vi "GOOP_MyComputer_Item_OnCommand.vi"(10 "Command Tag":string, 11 "Object":u64) -> ()   [LabVIEW 2012]
uses:
  <resource>/Framework/Providers/Open_GDS/SubVIs/GOOP_UMLEditor_CallMainAction.ctl
  <resource>/Framework/Providers/Open_GDS/ClassProviders/Provider_BaseClassInterface/ClassWriter_class/ClassWriter.lvclass
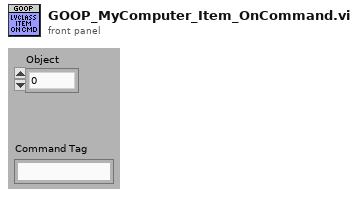
[diagram p1: front panel]
types:
  T1 = typedef "GOOP_UMLEditor_CallMainAction.ctl" = enum16{"OpenUmlEditor", "ReverseEngineering:WholeProject", "ReverseEngineering:OneClass", "ReverseEngineering:OneVI", "ShowInStateDiagram:OneVI", "OpenUMLFile"}
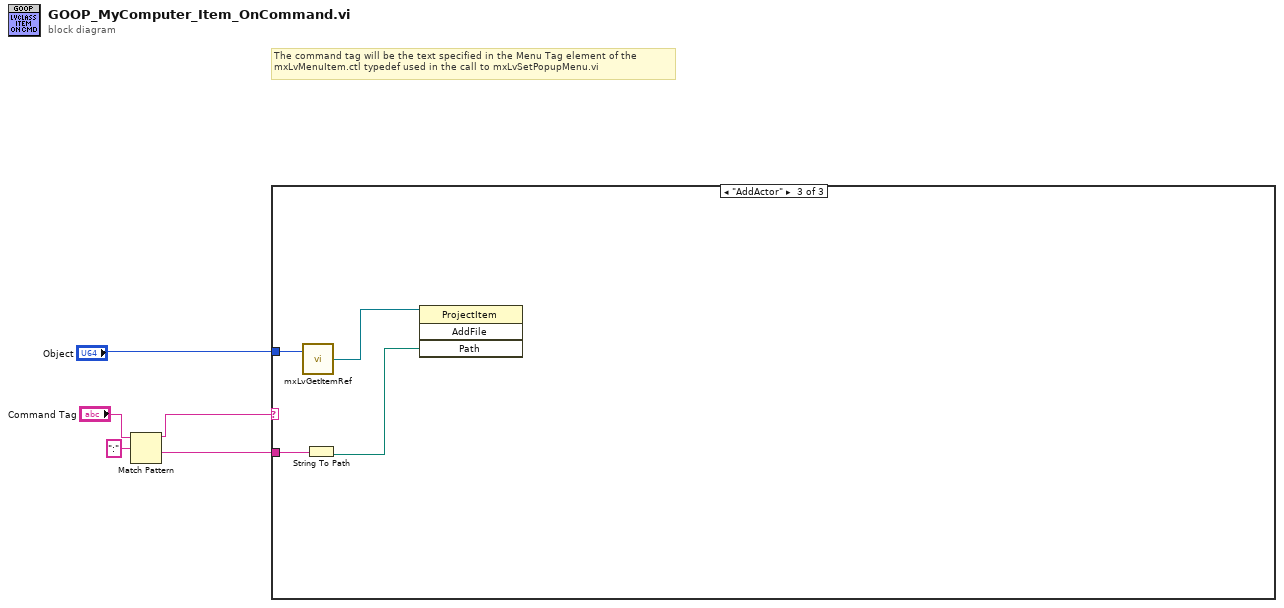
[diagram p0: block diagram]
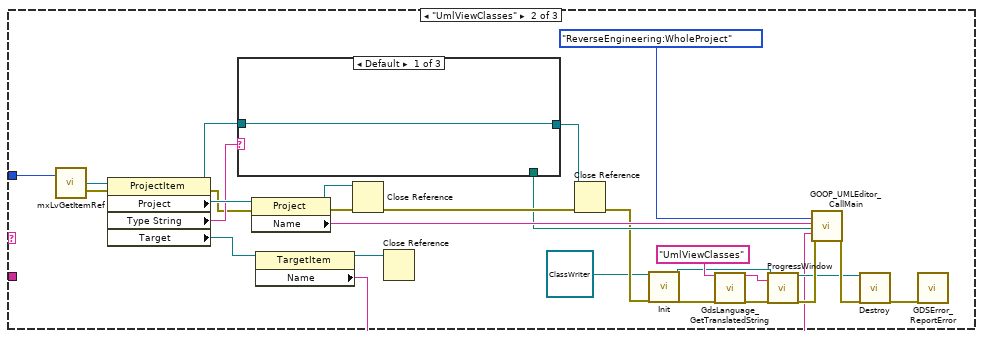
[diagram p3: hidden frame]
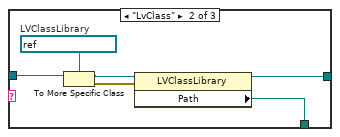
[diagram p4: hidden frame]
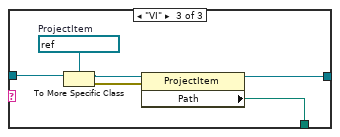
[diagram p5: hidden frame]
diagram:
  # "The command tag will be the text specified in the Menu Tag element of the \nmxLvMenuItem.ctl typedef used in the call to mxLvSetPopupMenu.vi"
  n1 = Match Pattern(string="Command Tag", regular expression=":") -> (before substring=w2:string, after substring=w1:string)  [unwired: 1 in, 2 out]
  n2 = case shown="\"AddActor\"" w2 {
    tunnel: "Object" -> [_ w32 w49]
    tunnel: w1 -> [_ _ w50]
    frame "False", Default {
    }
    frame "UmlViewClasses" {
      n3 = call <resource>:"mxLvGetItemRef.vi"("Item"=w32) -> ("Item Refnum"=w31:refnum<vi>, "error out"=w20:errorcluster)  [unwired: 1 in, 1 out]
      n4 = property class="ProjectItem"(reference=w31, error in=w20) -> (reference out=w25:refnum<vi>, error out=w21:errorcluster, "Project"=w30:refnum<vi>, "Type String"=w23:string, "Target"=w7:refnum<vi>)
      n5 = case shown="Default" w23 {
        tunnel: w25 -> [w34 w40 w46]
        tunnel: [w34 w36 w42] -> w24
        tunnel: [_ w35 w41] -> w22
        frame Default {
        }
        frame "LvClass" {
          w39 = refnum<vi> refnum  # LVClassLibrary
          n6 = To More Specific Class(target class=w39, reference=w40) -> (specific class reference=w38:refnum<vi>, error out=w37:errorcluster)  [unwired: 1 in]
          n7 = property class="LVClassLibrary"(reference=w38, error in=w37) -> (reference out=w36:refnum<vi>, "Path"=w35:path)  [unwired: 1 out]
        }
        frame "VI" {
          w45 = refnum<vi> refnum  # ProjectItem
          n8 = To More Specific Class(target class=w45, reference=w46) -> (specific class reference=w44:refnum<vi>, error out=w43:errorcluster)  [unwired: 1 in]
          n9 = property class="ProjectItem"(reference=w44, error in=w43) -> (reference out=w42:refnum<vi>, "Path"=w41:path)  [unwired: 1 out]
        }
      }
      n10 = property class="Project"(reference=w30, error in=w21) -> (reference out=w27:refnum<vi>, error out=w28:errorcluster, "Name"=w29:string)
      n11 = property class="TargetItem"(reference=w7) -> (reference out=w8:refnum<vi>, "Name"=w6:string)  [unwired: 1 in, 1 out]
      n12 = Close Reference(reference=w27, error in (no error)=w28) -> (error out=w26:errorcluster)
      n13 = Close Reference(reference=w8) -> ()  [unwired: 1 in, 1 out]
      n14 = Close Reference(reference=w24, error in (no error)=w26) -> (error out=w16:errorcluster)
      n15 = call-dynamic "Init.vi"("ClassWriter in"=refnum<class "ClassWriter.lvclass"> refnum, "error in (no error)"=w16) -> ("ClassWriter out"=w11:refnum<class "ClassWriter.lvclass">, "error out"=w15:errorcluster)  [unwired: 16 in]
      n16 = call <resource>:"GdsLanguage_GetTranslatedString.vi"("StringID(s)"="UmlViewClasses" ("Message(Exit)"), "error in (no error)"=w15) -> ("FirstStringOut"=w19:string, "error out"=w18:errorcluster)  [unwired: 14 in, 2 out]
      n17 = call-dynamic "ProgressWindow.vi"("ClassWriter in"=w11, "Message(Exit)"=w19, "error in (no error)"=w18) -> ("ClassWriter out"=w12:refnum<class "ClassWriter.lvclass">, "error out"=w14:errorcluster)  [unwired: 15 in]
      n18 = call <resource>:"GOOP_UMLEditor_CallMain.vi"("Enum"=GOOP_UMLEditor_CallMainAction."ReverseEngineering:WholeProject", "Project"=w29, "Class/VI-Path"=w22, "Target"=w6, "error in (no error)"=w14) -> ("error out"=w13:errorcluster)  [unwired: 14 in]
      n19 = call-dynamic "Destroy.vi"("ClassWriter.lvclass"=w12, "error in (no error)"=w13) -> ("error out"=w10:errorcluster)  [unwired: 17 in]
      n20 = call <resource>:"GDSError_ReportError.vi"("error in (no error)"=w10) -> ()  [unwired: 18 in, 1 out]
    }
    frame "AddActor" {
      n21 = call <resource>:"mxLvGetItemRef.vi"("Item"=w49) -> ("Item Refnum"=w48:refnum<vi>)  [unwired: 1 in, 2 out]
      n22 = String To Path(string=w50) -> (path=w47:path)
      n23 = invoke class="ProjectItem" method="AddFile"(reference=w48, "Path"=w47) -> ()  [unwired: 2 in, 4 out]
    }
  }
